vi "QTrkCreate.vi"(4 "error in (no error)":errorcluster, 5 "CUDA device selection":T1(ring), 6 "ROI":i32, 7 "QTrk Settings":T3={"Image width"=150, "Image height"=150, "Number of threads (CPU based)"=-1, "CUDA Device"=-2, "COM Background correction factor"=0.0, "ZLUT MinRadius"=8.0, "ZLUT Radial sample density"=5.0, "ZLUT Angular sample density"=2.0, "ZLUT ROI Coverage"=0.7, "QI Iterations"=2, "QI MinRadius"=5.0, "QI Radial sample density"=2.0, "QI Angular sample density"=0.7, "QI ROI Coverage"=1.0, "QI Angular Step \nIteration Factor"=128.0, "XCOR Profile Length"=32, "XCOR Profile Width"=2, "XCOR Iterations"=1, "Gaussian 2D Fit Iterations"=6, "Gaussian 2D Sigma (pixels)"=3.0}) -> (0 "error out":errorcluster, 1 "warnings":string, 3 "QTrk Instance":T2)   [LabVIEW 2011]
uses:
  QTrkSettings.ctl
  QTrkInstance.ctl
  QTrkDLL.vi
panel:
  out "return type":i64
  # "-2: Use all devices\n-1: Use best device"
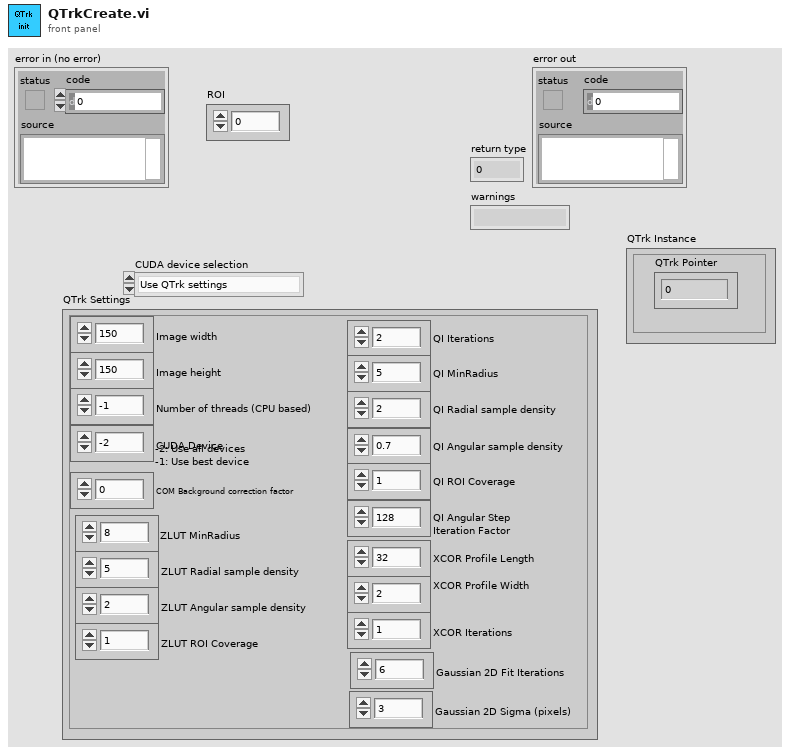
[diagram p1: front panel]
types:
  T1 = enum16{"Use QTrk settings", "Select best device", "Use all devices", "Use custom list"}
  T2 = typedef "QTrkInstance.ctl" = cluster{"QTrk Pointer":u64}
  T3 = typedef "QTrkSettings.ctl" = cluster{"Image width":i32, "Image height":i32, "Number of threads (CPU based)":i32, "CUDA Device":i32, "COM Background correction factor":sgl, "ZLUT MinRadius":sgl, "ZLUT Radial sample density":sgl, "ZLUT Angular sample density":sgl, "ZLUT ROI Coverage":sgl, "QI Iterations":i32, "QI MinRadius":sgl, "QI Radial sample density":sgl, "QI Angular sample density":sgl, "QI ROI Coverage":sgl, "QI Angular Step \nIteration Factor":sgl, "XCOR Profile Length":i32, "XCOR Profile Width":i32, "XCOR Iterations":i32, "Gaussian 2D Fit Iterations":i32, "Gaussian 2D Sigma (pixels)":sgl}
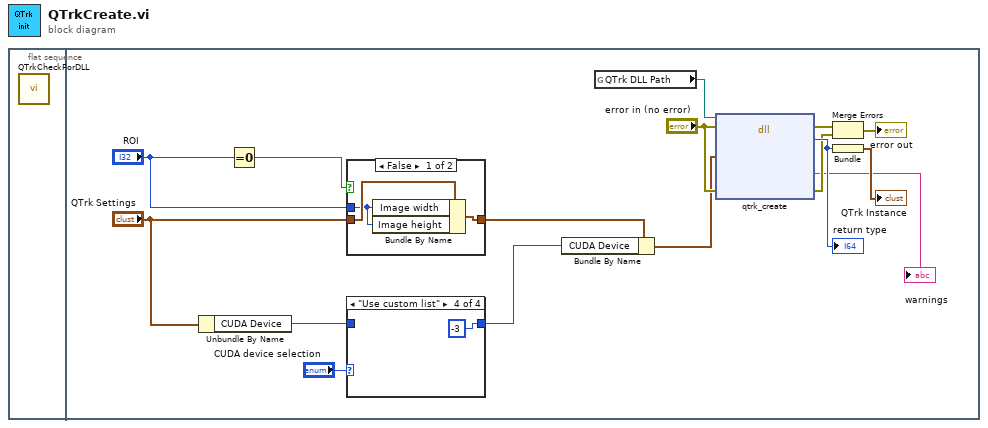
[diagram p0: block diagram]
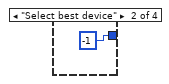
[diagram p3: hidden frame]
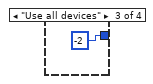
[diagram p4: hidden frame]
diagram:
  n1 = flat-sequence {
    frame #0 {
      n2 = call "QTrkCheckForDLL.vi"() -> ()  [unwired: 12 in]
    }
    frame #1 {
      n3 = Unbundle By Name("QTrk Settings") -> ("CUDA Device"=w2:i32)
      n4 = Equal To 0?(x="ROI") -> (x = 0?=w13:bool)
      n5 = case shown="False" w13 {
        tunnel: "QTrk Settings" -> [w23 w24]
        tunnel: [w22 w24] -> w6
        tunnel: "ROI" -> [w21 _]
        frame False {
          n6 = Bundle By Name(cluster=w23, "Image width"=w21, "Image height"=w21) -> (w22:T3)
        }
        frame True {
        }
      }
      n7 = case shown="\"Use custom list\"" "CUDA device selection" {
        tunnel: [w17 -1 -2 -3] -> w4
        tunnel: w2 -> [w17 _ _ _]
        frame "Use QTrk settings", Default {
        }
        frame "Select best device" {
        }
        frame "Use all devices" {
        }
        frame "Use custom list" {
        }
      }
      n8 = Bundle By Name(cluster=w6, "CUDA Device"=w4) -> (w5:T3)
      n9 = global read "QTrkDLL.vi" "QTrk DLL Path"() -> (w16:path)
      n10 = dll-call lib="F:/dev/jtrk/bin/jtrkd-labview-nt.dll" fn="qtrk_create"(path in=w16, error in="error in (no error)", "settings"=w5, "error"="error in (no error)") -> (error out=w10:errorcluster, "return type"=w15:u64, "warnings"=→"warnings":string, "error"=w9:errorcluster)  [unwired: 3 in, 1 out]
      "return type" <- w15
      n11 = Merge Errors(w10, w9) -> (→"error out":errorcluster)
      n12 = Bundle("return type"=w15) -> (→"QTrk Instance":cluster{"return type":u64})  [unwired: 1 in]
    }
  }
